vi "PH_PILS.PC _Experiment.vi"(0 "i ref in":refnum<vi>, 2 "Servicename":string, 3 "Value":i32, 5 "error IO":errorcluster) -> (14 "i ref out":refnum<vi>, 19 "error out":errorcluster)   [LabVIEW 2014, in "PH_PILS.lvlib"]
doc: "This VI writes incoming Tag datsa to own attributes."
uses:
  PH_PILS.lvlib
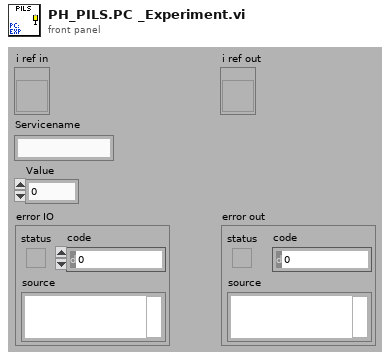
[diagram p1: front panel]
types:
  T1 = typedef "PH_PILS.lvlib/PH_PILS.i attribute.ctl" = cluster{"Boolean":cluster{"GUI Ref":refnum<vi>, "Status":i32}[], "GUI Refs Exp. Shutters":cluster{"1":refnum<vi>, "2":refnum<vi>, "3":refnum<vi>, "4":refnum<vi>}, "Tristate2Run GUI Refs":refnum<vi>[], "EO-Likes":cluster{"GUI Ref":refnum<vi>, "Status":i32}[], "Operation Mode":cluster{"Operation Mode":T2, "GUI":cluster{"Ref State":refnum<vi>, "Ref":refnum<vi>}, "Servicemode":cluster{"Tagname":string, "Status":i32}, "Labormode":cluster{"Tagname":string, "Status":i32}, "Searchmode":cluster{"Tagname":string, "Status":i32}, "Shotmode":cluster{"Tagname":string, "Status":i32}}, "Submode":cluster{"Submode":T3, "GUI":cluster{"Ref State":refnum<vi>, "Ref":refnum<vi>}, "Submode":cluster{"Tagname":string, "Status":i32}}, "Experiment":cluster{"Experiment":enum16{"unknown", "intern", "4 (Z6)", "3", "2", "1"}, "GUI":cluster{"Ref State":refnum<vi>, "Ref":refnum<vi>}, "intern":cluster{"Tagname":string, "Status":i32}, "Exp 4":cluster{"Tagname":string, "Status":i32}, "Exp 3":cluster{"Tagname":string, "Status":i32}, "Exp 2":cluster{"Tagname":string, "Status":i32}, "Exp 1":cluster{"Tagname":string, "Status":i32}}, "TristateNormal":cluster{"GUI Ref":refnum<vi>, "Status":i32}[], "Door Tags":cluster{"GUI Ref":refnum<vi>, "Status":i32}[], "GUIlessTags":cluster{"Name":string, "Status":i32}[], "Beamline GUI Refs":refnum<vi>[], "Special Boolean":cluster{"GUI Ref":refnum<vi>, "Status":i32}[], "Laserpower":cluster{"GUI Ref":refnum<vi>, "Status":i32}[], "Shutter":cluster{"GUI Ref":refnum<vi>, "Status":i32}[], "Tristate EO Like":cluster{"GUI Ref":refnum<vi>, "Status":i32}[], "PP":cluster{"GUI Ref":refnum<vi>, "Status":i32, "Head Ref":refnum<vi>, "Slider Ref":refnum<vi>}[], "Switch Knobs":cluster{"GUI Ref":refnum<vi>, "Status":i32}[], "Latch Knob GUI Refs":refnum<vi>[], "FailureCounter":i32, "Enabled Status":cluster{"Laser":i32, "PreAmp":i32, "MainAmp":i32}, "Mercury":refnum<vi>, "Instance Rods":string, "Logfile":path, "Beckhoff-Instance Internal":string, "Beckhoff-Instance External":string, "Enabling Rights":cluster{"Name":string, "Password":string, "PA?":bool, "MA?":bool, "Exp?":bool}[]}
  T2 = typedef "PH_PILS.lvlib/PH_PILS.Operation Mode.ctl" = enum16{"unknown", "Service", "Labor", "Search", "Shot"}
  T3 = typedef "PH_PILS.lvlib/PH_PILS.Submode.ctl" = enum16{"unknown", "HV-Normal", "HV-Test"}
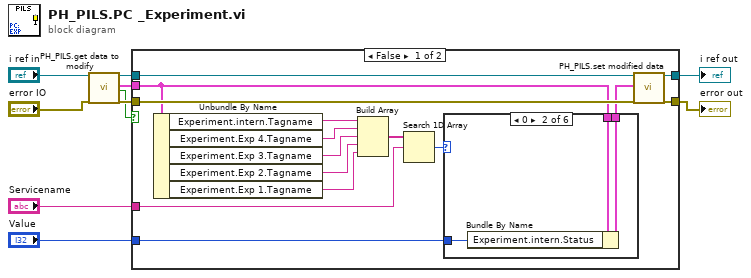
[diagram p0: block diagram]
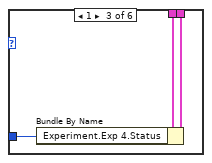
[diagram p3: hidden frame]
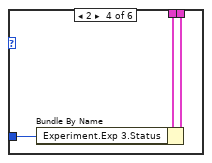
[diagram p4: hidden frame]
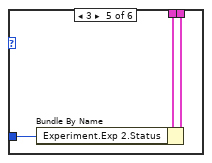
[diagram p5: hidden frame]
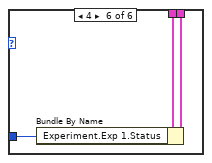
[diagram p6: hidden frame]
diagram:
  n1 = call "PH_PILS.get data to modify.vi"("i ref in"="i ref in", "error in (no error)"="error IO") -> ("i ref out"=w9:refnum<vi>, "i attribute"=w5:T1, "timed out"=w6:bool, "error out"=w10:errorcluster)  [unwired: 14 in]
  n2 = case shown="False" w6 {
    tunnel: [w25 w42] -> w1
    tunnel: w10 -> [w24 w42]
    tunnel: [w23 w43] -> w2
    tunnel: w9 -> [w22 w43]
    tunnel: w5 -> [w15 _]
    tunnel: "Servicename" -> [w16 _]
    tunnel: "Value" -> [w12 _]
    frame False {
      n3 = Unbundle By Name(w15) -> ("Experiment.intern.Tagname"=w21:string, "Experiment.Exp 4.Tagname"=w20:string, "Experiment.Exp 3.Tagname"=w19:string, "Experiment.Exp 2.Tagname"=w18:string, "Experiment.Exp 1.Tagname"=w11:string)
      n4 = Build Array(w21, w20, w19, w18, w11) -> (w17:string[])
      n5 = Search 1D Array(1D array=w17, element=w16) -> (index of element=w14:i32)  [unwired: 1 in]
      n6 = case shown="0" w14 {
        tunnel: w15 -> [w26 w29 w32 w35 w38 w41]
        tunnel: [w26 w28 w31 w34 w37 w40] -> w13
        tunnel: w12 -> [_ w27 w30 w33 w36 w39]
        frame Default {
        }
        frame 0 {
          n7 = Bundle By Name(cluster=w29, "Experiment.intern.Status"=w27) -> (w28:T1)
        }
        frame 1 {
          n8 = Bundle By Name(cluster=w32, "Experiment.Exp 4.Status"=w30) -> (w31:T1)
        }
        frame 2 {
          n9 = Bundle By Name(cluster=w35, "Experiment.Exp 3.Status"=w33) -> (w34:T1)
        }
        frame 3 {
          n10 = Bundle By Name(cluster=w38, "Experiment.Exp 2.Status"=w36) -> (w37:T1)
        }
        frame 4 {
          n11 = Bundle By Name(cluster=w41, "Experiment.Exp 1.Status"=w39) -> (w40:T1)
        }
      }
      n12 = call "PH_PILS.set modified data.vi"("i ref in"=w22, "i attribute"=w13, "error in (no error)"=w24) -> ("i ref out"=w23:refnum<vi>, "error out"=w25:errorcluster)  [unwired: 15 in]
    }
    frame True {
    }
  }
  "error out" <- w1
  "i ref out" <- w2
